vi "STATus.vi"(8 "Error in (no error)":errorcluster, 9 "Enable":u16 format="%04x", 10 "Function":T1(ring), 11 "VISA resource":refnum<visa-resource-name>) -> (0 "Error out":errorcluster, 1 "Enable out":i32 format="%04x", 2 "Response":string, 3 "Dup VISA resource":refnum<visa-resource-name>)   [LabVIEW 2010]
doc: "Copyright (c) 2012 Metrolab Technology SA, Plan-les-Ouates, Geneva, Switzerland\nCollects all commands concerning the IEEE488.2 / SCPI status system in the THM116. See the manual for more details about the status registers."
panel:
  # "STATus"
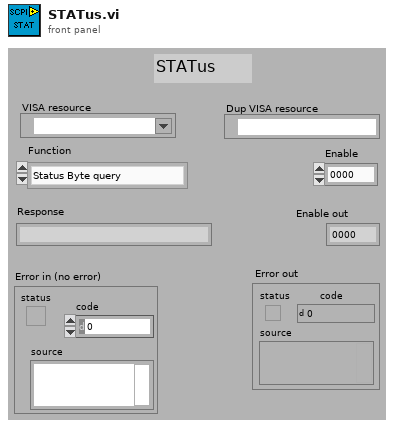
[diagram p1: front panel]
types:
  T1 = enum16{"Status Byte query", "Status Enable query", "Status Enable", "Event Status query", "Event Enable query", "Event Enable", "OPER EVENt query", "OPER CONDition query", "OPER ENABle query", "OPER ENABle", "QUES EVENt query", "QUES CONDition query", "QUES ENABle query", "QUES ENABle", "Error/Event Queue query", "Clear Status", "PRESet"}
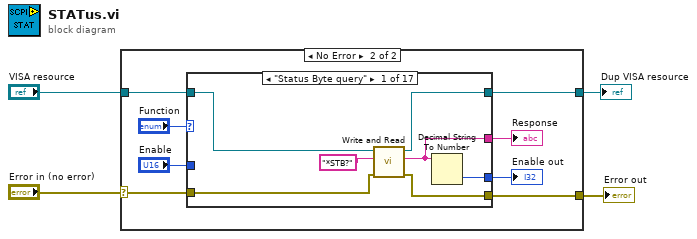
[diagram p0: block diagram]
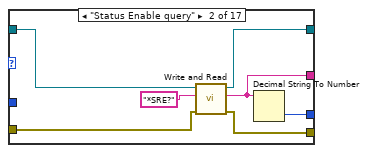
[diagram p3: hidden frame]
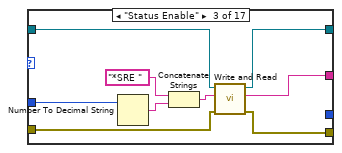
[diagram p4: hidden frame]
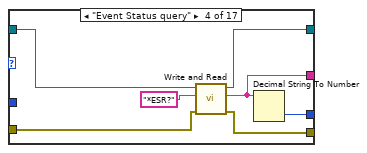
[diagram p5: hidden frame]
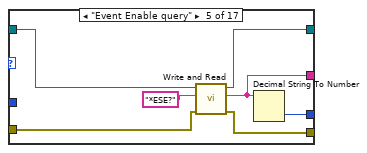
[diagram p6: hidden frame]
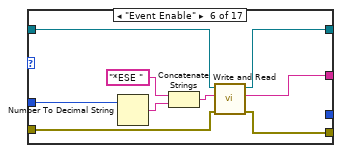
[diagram p7: hidden frame]
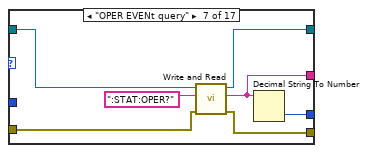
[diagram p8: hidden frame]
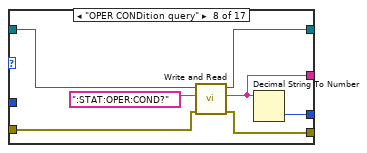
[diagram p9: hidden frame]
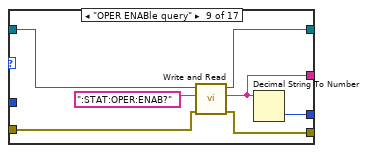
[diagram p10: hidden frame]
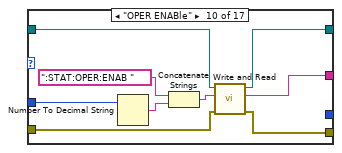
[diagram p11: hidden frame]
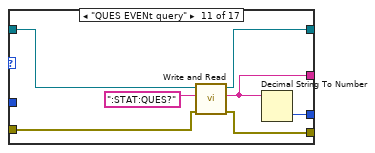
[diagram p12: hidden frame]
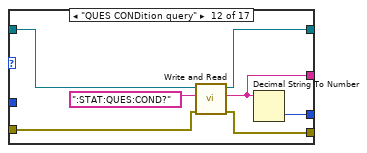
[diagram p13: hidden frame]
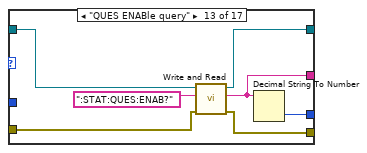
[diagram p14: hidden frame]
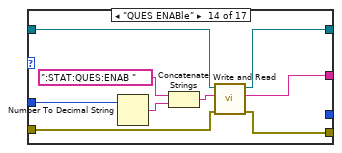
[diagram p15: hidden frame]
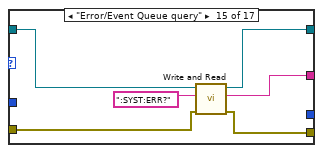
[diagram p16: hidden frame]
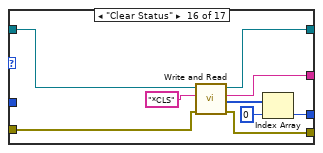
[diagram p17: hidden frame]
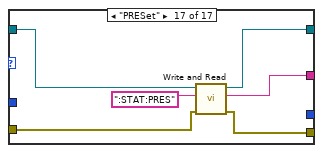
[diagram p18: hidden frame]
diagram:
  n1 = case shown="No Error" "Error in (no error)" {
    selector: "Error in (no error)" -> [w5 w12]
    tunnel: "VISA resource" -> [w6 w13]
    tunnel: [w6 w11] -> w1
    tunnel: [w5 w10] -> w4
    frame Error {
    }
    frame No Error {
      n2 = case shown="\"Status Byte query\"" "Function" {
        tunnel: w13 -> [w21 w28 w34 w44 w51 w57 w67 w74 w81 w87 w97 w104 w111 w117 w126 w134 w141]
        tunnel: w12 -> [w20 w27 w35 w43 w45 w58 w66 w73 w80 w88 w91 w103 w110 w118 w125 w133 w140]
        tunnel: [w19 w26 w33 w42 w50 w56 w65 w72 w79 w86 w96 w102 w109 w116 w122 w130 w137] -> w11
        tunnel: [w18 w25 w32 w41 w49 w55 w64 w71 w78 w85 w95 w101 w108 w115 w123 w131 w138] -> w10
        tunnel: [w17 w24 w31 w40 w48 w54 w63 w70 w77 w84 w94 w100 w107 w114 w124 w132 w139] -> w9
        tunnel: [w16 w23 _ w39 w47 _ w62 w69 w76 _ w93 w99 w106 _ _ w127 _] -> w8
        tunnel: "Enable" -> [_ _ w30 _ _ w53 _ _ _ w83 _ _ _ w113 _ _ _]
        frame "Status Byte query" {
          n3 = call "Write and Read.vi"("Error in (no error)"=w20, "Command"="*STB?", "VISA resource"=w21) -> ("Error out"=w18:errorcluster, "Response"=w17:string, "Dup VISA resource"=w19:refnum<visa-resource-name>)  [unwired: 4 in, 2 out]
          n4 = Decimal String To Number(string=w17) -> (number=w16:i32)  [unwired: 2 in, 1 out]
        }
        frame "Status Enable query" {
          n5 = call "Write and Read.vi"("Error in (no error)"=w27, "Command"="*SRE?", "VISA resource"=w28) -> ("Error out"=w25:errorcluster, "Response"=w24:string, "Dup VISA resource"=w26:refnum<visa-resource-name>)  [unwired: 4 in, 2 out]
          n6 = Decimal String To Number(string=w24) -> (number=w23:i32)  [unwired: 2 in, 1 out]
        }
        frame "Status Enable" {
          n7 = Number To Decimal String(number=w30) -> (decimal integer string=w37:string)  [unwired: 1 in]
          n8 = Concatenate Strings("*SRE " ("string"), w37) -> (w36:string)
          n9 = call "Write and Read.vi"("Error in (no error)"=w35, "Command"=w36, "VISA resource"=w34) -> ("Error out"=w32:errorcluster, "Response"=w31:string, "Dup VISA resource"=w33:refnum<visa-resource-name>)  [unwired: 4 in, 2 out]
        }
        frame "Event Status query" {
          n10 = call "Write and Read.vi"("Error in (no error)"=w43, "Command"="*ESR?", "VISA resource"=w44) -> ("Error out"=w41:errorcluster, "Response"=w40:string, "Dup VISA resource"=w42:refnum<visa-resource-name>)  [unwired: 4 in, 2 out]
          n11 = Decimal String To Number(string=w40) -> (number=w39:i32)  [unwired: 2 in, 1 out]
        }
        frame "Event Enable query" {
          n12 = call "Write and Read.vi"("Error in (no error)"=w45, "Command"="*ESE?", "VISA resource"=w51) -> ("Error out"=w49:errorcluster, "Response"=w48:string, "Dup VISA resource"=w50:refnum<visa-resource-name>)  [unwired: 4 in, 2 out]
          n13 = Decimal String To Number(string=w48) -> (number=w47:i32)  [unwired: 2 in, 1 out]
        }
        frame "Event Enable" {
          n14 = Number To Decimal String(number=w53) -> (decimal integer string=w60:string)  [unwired: 1 in]
          n15 = Concatenate Strings("*ESE " ("string"), w60) -> (w59:string)
          n16 = call "Write and Read.vi"("Error in (no error)"=w58, "Command"=w59, "VISA resource"=w57) -> ("Error out"=w55:errorcluster, "Response"=w54:string, "Dup VISA resource"=w56:refnum<visa-resource-name>)  [unwired: 4 in, 2 out]
        }
        frame "OPER EVENt query" {
          n17 = call "Write and Read.vi"("Error in (no error)"=w66, "Command"=":STAT:OPER?", "VISA resource"=w67) -> ("Error out"=w64:errorcluster, "Response"=w63:string, "Dup VISA resource"=w65:refnum<visa-resource-name>)  [unwired: 4 in, 2 out]
          n18 = Decimal String To Number(string=w63) -> (number=w62:i32)  [unwired: 2 in, 1 out]
        }
        frame "OPER CONDition query" {
          n19 = call "Write and Read.vi"("Error in (no error)"=w73, "Command"=":STAT:OPER:COND?", "VISA resource"=w74) -> ("Error out"=w71:errorcluster, "Response"=w70:string, "Dup VISA resource"=w72:refnum<visa-resource-name>)  [unwired: 4 in, 2 out]
          n20 = Decimal String To Number(string=w70) -> (number=w69:i32)  [unwired: 2 in, 1 out]
        }
        frame "OPER ENABle query" {
          n21 = call "Write and Read.vi"("Error in (no error)"=w80, "Command"=":STAT:OPER:ENAB?", "VISA resource"=w81) -> ("Error out"=w78:errorcluster, "Response"=w77:string, "Dup VISA resource"=w79:refnum<visa-resource-name>)  [unwired: 4 in, 2 out]
          n22 = Decimal String To Number(string=w77) -> (number=w76:i32)  [unwired: 2 in, 1 out]
        }
        frame "OPER ENABle" {
          n23 = Number To Decimal String(number=w83) -> (decimal integer string=w90:string)  [unwired: 1 in]
          n24 = Concatenate Strings(":STAT:OPER:ENAB " ("string"), w90) -> (w89:string)
          n25 = call "Write and Read.vi"("Error in (no error)"=w88, "Command"=w89, "VISA resource"=w87) -> ("Error out"=w85:errorcluster, "Response"=w84:string, "Dup VISA resource"=w86:refnum<visa-resource-name>)  [unwired: 4 in, 2 out]
        }
        frame "QUES EVENt query" {
          n26 = call "Write and Read.vi"("Error in (no error)"=w91, "Command"=":STAT:QUES?", "VISA resource"=w97) -> ("Error out"=w95:errorcluster, "Response"=w94:string, "Dup VISA resource"=w96:refnum<visa-resource-name>)  [unwired: 4 in, 2 out]
          n27 = Decimal String To Number(string=w94) -> (number=w93:i32)  [unwired: 2 in, 1 out]
        }
        frame "QUES CONDition query" {
          n28 = call "Write and Read.vi"("Error in (no error)"=w103, "Command"=":STAT:QUES:COND?", "VISA resource"=w104) -> ("Error out"=w101:errorcluster, "Response"=w100:string, "Dup VISA resource"=w102:refnum<visa-resource-name>)  [unwired: 4 in, 2 out]
          n29 = Decimal String To Number(string=w100) -> (number=w99:i32)  [unwired: 2 in, 1 out]
        }
        frame "QUES ENABle query" {
          n30 = call "Write and Read.vi"("Error in (no error)"=w110, "Command"=":STAT:QUES:ENAB?", "VISA resource"=w111) -> ("Error out"=w108:errorcluster, "Response"=w107:string, "Dup VISA resource"=w109:refnum<visa-resource-name>)  [unwired: 4 in, 2 out]
          n31 = Decimal String To Number(string=w107) -> (number=w106:i32)  [unwired: 2 in, 1 out]
        }
        frame "QUES ENABle" {
          n32 = Number To Decimal String(number=w113) -> (decimal integer string=w120:string)  [unwired: 1 in]
          n33 = Concatenate Strings(":STAT:QUES:ENAB " ("string"), w120) -> (w119:string)
          n34 = call "Write and Read.vi"("Error in (no error)"=w118, "Command"=w119, "VISA resource"=w117) -> ("Error out"=w115:errorcluster, "Response"=w114:string, "Dup VISA resource"=w116:refnum<visa-resource-name>)  [unwired: 4 in, 2 out]
        }
        frame "Error/Event Queue query" {
          n35 = call "Write and Read.vi"("Error in (no error)"=w125, "Command"=":SYST:ERR?", "VISA resource"=w126) -> ("Error out"=w123:errorcluster, "Response"=w124:string, "Dup VISA resource"=w122:refnum<visa-resource-name>)  [unwired: 4 in, 2 out]
        }
        frame "Clear Status" {
          n36 = call "Write and Read.vi"("Error in (no error)"=w133, "Command"="*CLS", "VISA resource"=w134) -> ("Error out"=w131:errorcluster, "Response"=w132:string, "Dup VISA resource"=w130:refnum<visa-resource-name>, "Status Bytes"=w135:u16[])  [unwired: 4 in, 1 out]
          n37 = Index Array(array=w135, index=0) -> (element=w127:u16)
        }
        frame "PRESet" {
          n38 = call "Write and Read.vi"("Error in (no error)"=w140, "Command"=":STAT:PRES", "VISA resource"=w141) -> ("Error out"=w138:errorcluster, "Response"=w139:string, "Dup VISA resource"=w137:refnum<visa-resource-name>)  [unwired: 4 in, 2 out]
        }
      }
      "Response" <- w9
      "Enable out" <- w8
    }
  }
  "Error out" <- w4
  "Dup VISA resource" <- w1
